vi "fpga main2.vi"() -> ()   [LabVIEW 2017]
uses:
  <vilib>/rvi/Emulation/niFpgaGetClockAttributes.vi
  <vilib>/rvi/Emulation/niFpgaSctlEmulationGetInTimedLoop.vi
  <vilib>/rvi/Emulation/niFpgaEmulationReportErrorSimple.vi
  <vilib>/rvi/eio/common/nirviEmuTemplateMethod_errors.vi
  <vilib>/rvi/interface/RandomDataEmulation/niFpgaRandomDataHandleErrors.vi
  <vilib>/rvi/Emulation/niFpgaCriticalErrorInLSC.vi
  <vilib>/eio/EIONode/EIONode.xnode
  <vilib>/rvi/Arithmetic/AddSubMult/XNode/nirviSatArithmetic.xnode
  <vilib>/rvi/DataTransferAndStorage/Container/XNode/niFpgaContainer.xnode
  <vilib>/rvi/interface/RandomDataEmulation/nirviRandomDataFpgaReadWriteTemplate.vi
panel:
  out "Timed Out?":bool
  out "real period":u32
  in  "Position Reset":bool
  in  "Velocity Interval (mSec)":u32=1000
  in  "stop 2":bool
  out "Position (Counts)":i32
  out "Acceleration (Counts/Interval)":i32
  out "Velocity (Counts/Interval)":i32
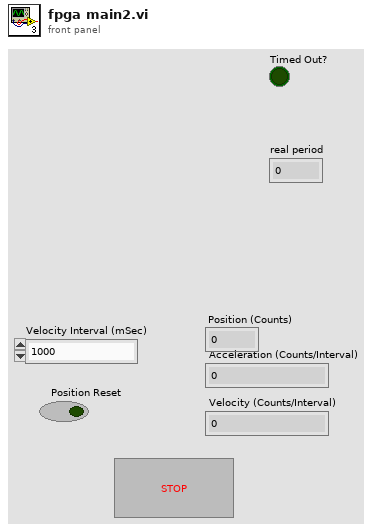
[diagram p1: front panel]
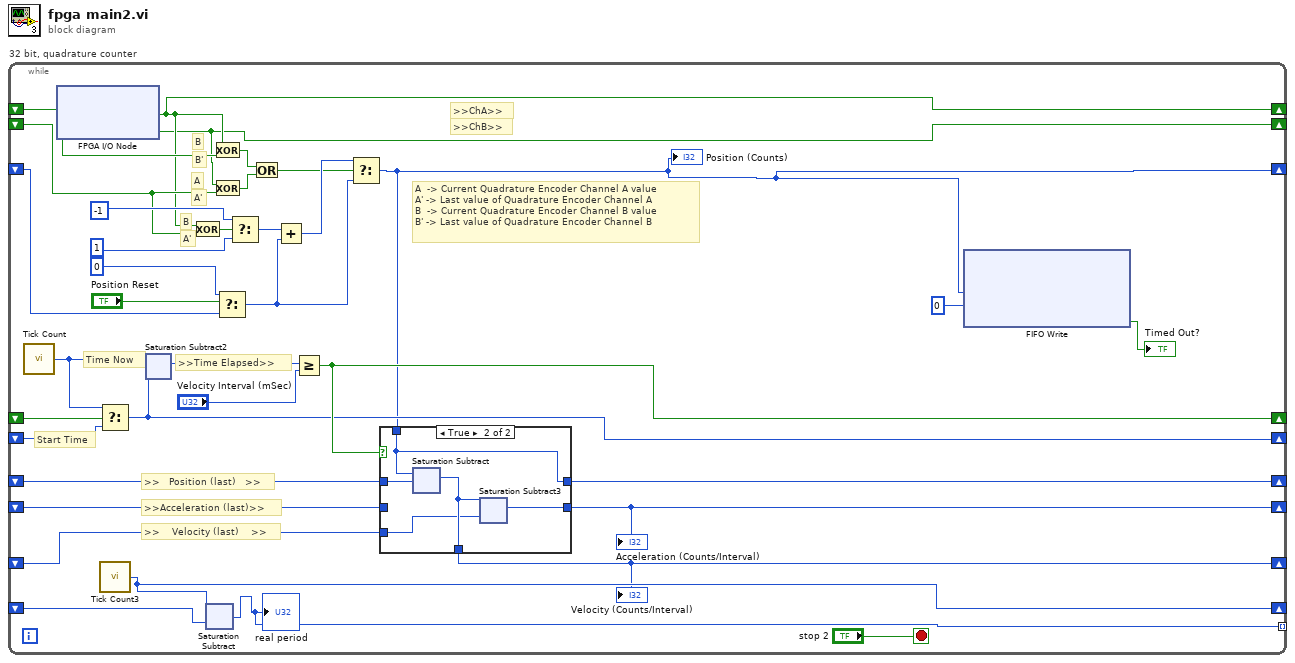
[diagram p0: block diagram]
diagram:
  n1 = while "32 bit, quadrature counter" {
    shift-right: [w11] -> _
    shift-left: _ -> [w12]
    shift-right: [w1] -> _
    shift-left: _ -> [w23]
    shift-right: [w10] -> _
    shift-left: _ -> [w26]
    shift-right: [w19] -> _
    shift-left: _ -> [w22]
    shift-right: [w14] -> _
    shift-left: _ -> [w20]
    shift-right: [w6] -> _
    shift-left: _ -> [w17]
    shift-right: [w5] -> _
    shift-left: _ -> [w16]
    shift-right: [w4] -> _
    shift-left: _ -> [w13]
    shift-right: [w9] -> _
    shift-left: _ -> [w8]
    tunnel: [w7] -> _ mode=indexing
    stop <- "stop 2" stop-if-true
    # "A  -> Current Quadrature Encoder Channel A value\nA' -> Last value of Quadrature Encoder Channel A\nB  -> Current Quadrature Encoder Channel B value\nB' -> Last value of Quadrature Encoder Channel B"
    # ">>Acceleration (last)>>"
    # "Start Time"
    # "A'"
    # "B"
    # "A'"
    # "A"
    # "B'"
    # "B"
    # ">>ChB>>"
    # ">>ChA>>"
    # ">>    Velocity (last)    >>"
    # ">>   Position (last)   >>"
    # "Time Now"
    # ">>Time Elapsed>>"
    n2 = call "Tick Count"() -> ("Tick Count(mSec)"=w15:u32)
    n3 = xnode "FPGA I/O Node"() -> ("Mod1/DI0"=w11:bool, "Mod1/DI1"=w10:bool)  [unwired: 2 in, 2 out]
    n4 = Select(t=w15, s=w22, f=w20) -> (s? t:f=w14:u32)
    n5 = call "Tick Count3"() -> ("Tick Count(uSec)"=w9:u32)
    n6 = xnode ("Saturation Subtract2")("x"=w15, "y"=w14) -> ("x-y"=w18:u32)
    n7 = Exclusive Or(1:w26, 2:w11) -> (0:w27:bool)
    n8 = xnode ("Saturation Subtract")("x"=w9, "y"=w8) -> ("x-y"=w7:u32)
    "real period" <- w7
    n9 = Exclusive Or(1:w12, 2:w11) -> (0:w28:bool)
    n10 = Exclusive Or(1:w26, 2:w10) -> (0:w29:bool)
    n11 = Select(t=0 ("32 bit"), s="Position Reset", f=w23) -> (s? t:f=w34:i32)
    n12 = Select(t=-1 ("32 bit"), s=w27, f=1 ("32 bit")) -> (s? t:f=w32:i32)
    n13 = Or(x=w28, y=w29) -> (x .or. y?=w24:bool)
    n14 = Add(x=w32, y=w34) -> (x+y=w36:i32)
    n15 = Greater Or Equal?(x=w18, y="Velocity Interval (mSec)") -> (x >= y?=w19:bool)
    n16 = Select(t=w36, s=w24, f=w34) -> (s? t:f=w1:i32)
    "Position (Counts)" <- w1
    n17 = case shown="True" w19 {
      tunnel: w1 -> [_ w60]
      tunnel: w17 -> [w57 w64]
      tunnel: [w59 w63] -> w5
      tunnel: w16 -> [w59 w62]
      tunnel: [w58 w61] -> w4
      tunnel: w13 -> [w58 _]
      tunnel: [w57 w60] -> w6
      frame False {
      }
      frame True {
        n18 = xnode ("Saturation Subtract")("x"=w60, "y"=w64) -> ("x-y"=w63:i32)
        n19 = xnode ("Saturation Subtract3")("x"=w63, "y"=w62) -> ("x-y"=w61:i32)
      }
    }
    "Acceleration (Counts/Interval)" <- w4
    "Velocity (Counts/Interval)" <- w5
    n20 = xnode ("FIFO Write")("Element"=w1, "Timeout"=0) -> ("Timed Out?"=→"Timed Out?":bool)  [unwired: 1 in, 1 out]
  }
